vi "Post-Build Action.vi"(5 "Files Generated by Build":path[](array[path]), 6 "Top Level/Always Included VIs":path[](array[path]), 7 "Destination Path":path, 8 "error in (no error)":errorcluster, 9 "Target Name":string, 10 "Build Specification Name":string, 11 "Project Path":path) -> (0 "error out":errorcluster)   [LabVIEW 2017]
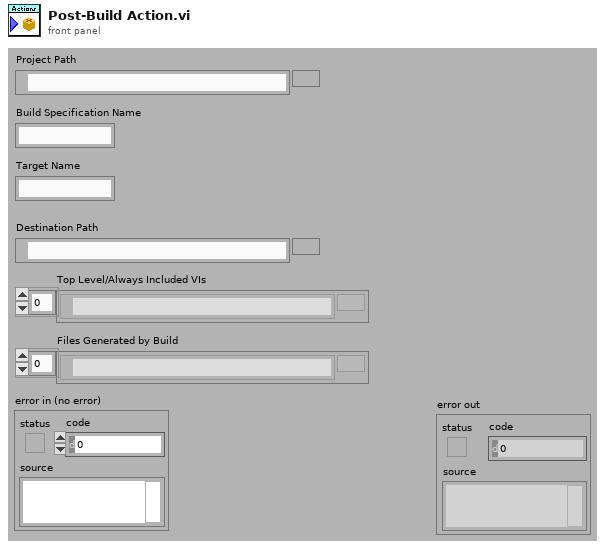
[diagram p1: front panel]
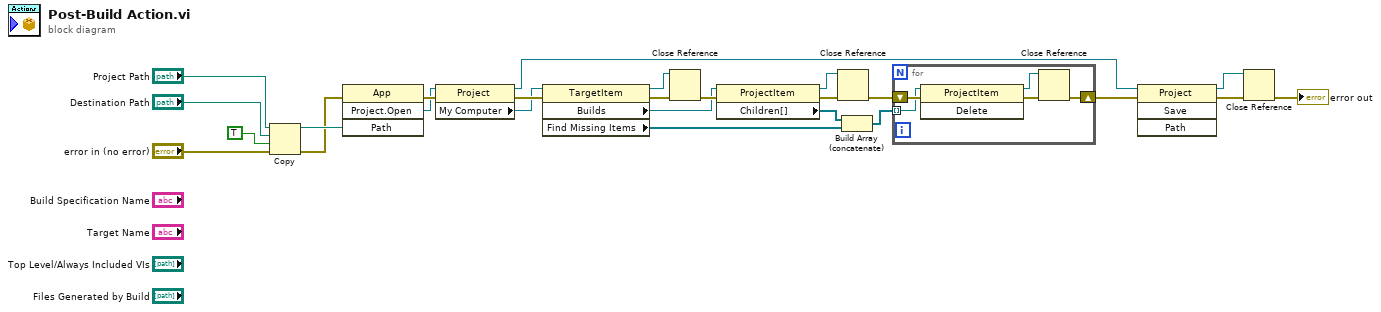
[diagram p0: block diagram]
diagram:
  n1 = Copy(8:"error in (no error)", 9:TRUE ("overwrite (F)"), 10:"Destination Path", 11:"Project Path") -> (0:w17:errorcluster, 3:w24:path)  [unwired: 1 in, 1 out]
  n2 = invoke class="App" method="Project.Open"(error in=w17, "Path"=w24) -> (error out=w21:errorcluster, "Project:Open"=w7:refnum<vi>)  [unwired: 2 in, 2 out]
  n3 = property class="Project"(reference=w7, error in=w21) -> (reference out=w23:refnum<vi>, error out=w22:errorcluster, "My Computer"=w5:refnum<vi>)
  n4 = property class="TargetItem"(reference=w5, error in=w22) -> (reference out=w9:refnum<vi>, error out=w10:errorcluster, "Builds"=w6:refnum<vi>, "Find Missing Items"=w3:refnum<vi>[])
  n5 = Close Reference(reference=w9, error in (no error)=w10) -> (error out=w8:errorcluster)
  n6 = property class="ProjectItem"(reference=w6, error in=w8) -> (reference out=w12:refnum<vi>, error out=w13:errorcluster, "Children[]"=w4:refnum<vi>[])
  n7 = Close Reference(reference=w12, error in (no error)=w13) -> (error out=w11:errorcluster)
  n8 = Build Array (concatenate)(w4, w3) -> (w2:refnum<vi>[])
  n9 = for {
    shift-right: [w27] -> w1
    shift-left: w11 -> [w30]
    tunnel: w2 -> [w29] mode=indexing
    n10 = invoke class="ProjectItem" method="Delete"(reference=w29, error in=w30) -> (reference out=w26:refnum<vi>, error out=w28:errorcluster)  [unwired: 1 in, 1 out]
    n11 = Close Reference(reference=w26, error in (no error)=w28) -> (error out=w27:errorcluster)
  }
  n12 = invoke class="Project" method="Save"(reference=w23, error in=w1) -> (reference out=w14:refnum<vi>, error out=w16:errorcluster)  [unwired: 2 in, 2 out]
  n13 = Close Reference(reference=w14, error in (no error)=w16) -> (error out=→"error out":errorcluster)
